vi "Stimulus trigger logic-Funct protocols.vi"(8 "Start trigger not fired":bool, 9 "Trigger lines value":T1, 10 "Tick Count(Ticks) in":u32, 11 "Stimulus Trigger Setup":T2={"Trigger period in live protocols (80MHz Cycles)"=510000000, "Pulse width in live protocols (80MHz Cycles)"=80000000, "Enable stimulus in live protocols"=FALSE, "Trigger delay in funct. protocols (80MHz Cycles)"=0, "Pulse width in funct. protocols (80MHz Cycles)"=400000, "Enable stimulus in funct. protocols"=FALSE}) -> (0 "Start trigger not fired":bool, 2 "Tick Count(Ticks) out":u32, 5 "Output value":bool)   [LabVIEW 2020]
uses:
  <vilib>/eio/EIONode/EIONode.xnode
  <vilib>/rvi/eio/common/nirviEmuTemplateMethod_errors.vi
  FPGA Typedefs/Stimulus trigger delays cluster.ctl
  FPGA Typedefs/PXI Trigger lines value cluster.ctl
panel:
  out "RAW counter VI":u32
  # "Limited to 53.5 sec (if U32)"
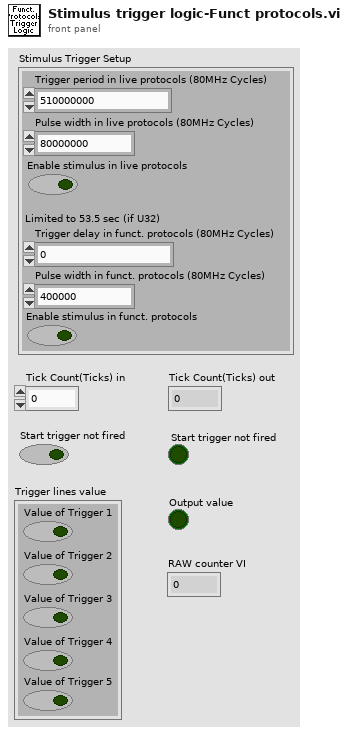
[diagram p1: front panel]
types:
  T1 = typedef "PXI Trigger lines value cluster.ctl" = cluster{"Value of Trigger 1":bool, "Value of Trigger 2":bool, "Value of Trigger 3":bool, "Value of Trigger 4":bool, "Value of Trigger 5":bool}
  T2 = typedef "Stimulus trigger delays cluster.ctl" = cluster{"Trigger period in live protocols (80MHz Cycles)":u32, "Pulse width in live protocols (80MHz Cycles)":u32, "Enable stimulus in live protocols":bool, "Trigger delay in funct. protocols (80MHz Cycles)":u32, "Pulse width in funct. protocols (80MHz Cycles)":u32, "Enable stimulus in funct. protocols":bool}
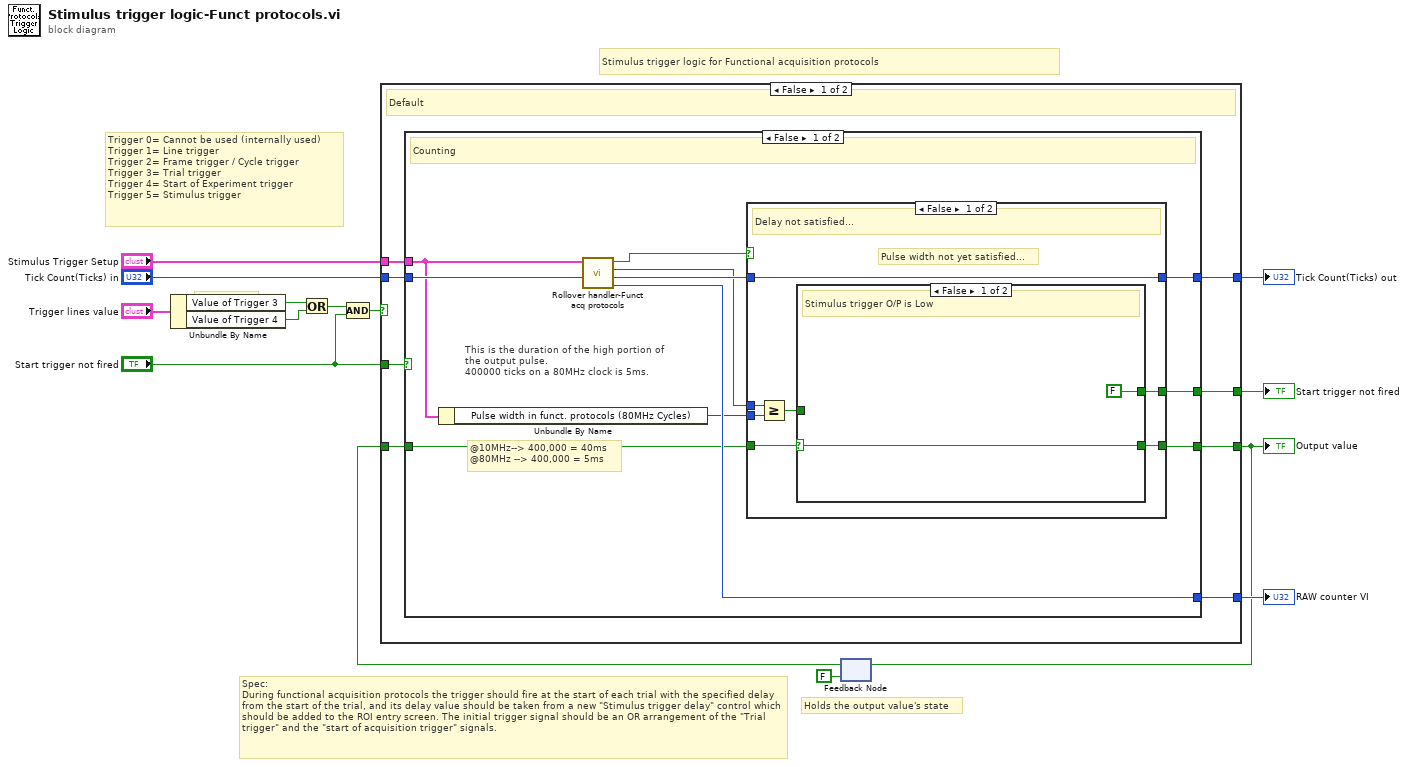
[diagram p0: block diagram]
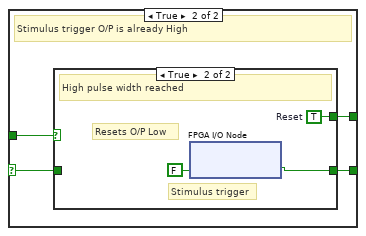
[diagram p2: hidden frame]
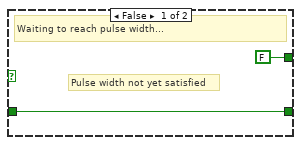
[diagram p3: hidden frame]
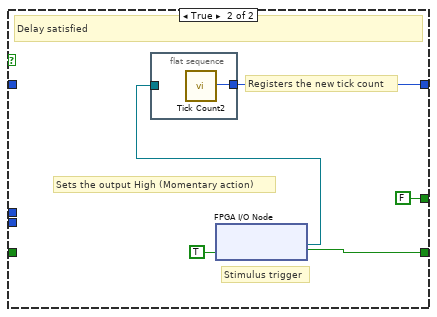
[diagram p4: hidden frame]
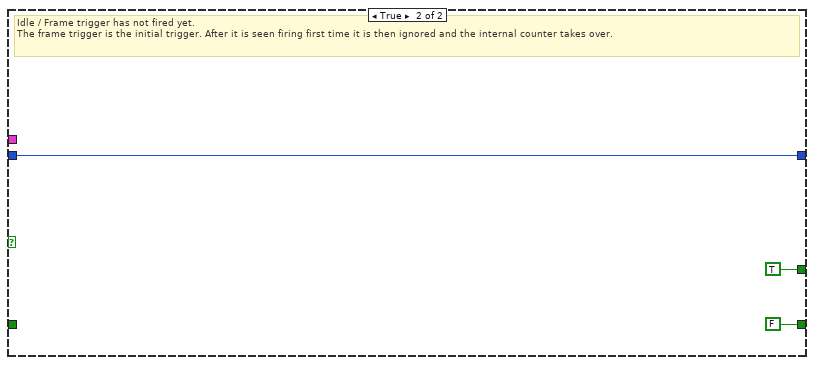
[diagram p5: hidden frame]
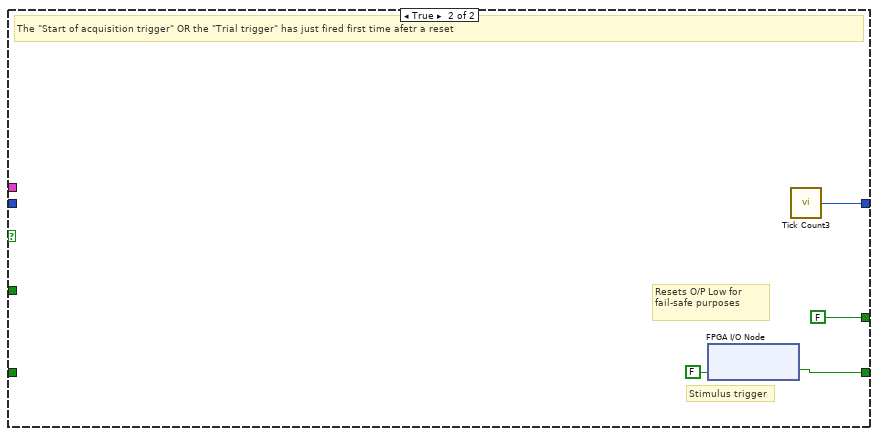
[diagram p6: hidden frame]
diagram:
  # "Holds the output value's state"
  # "Trigger 0= Cannot be used (internally used)\nTrigger 1= Line trigger\nTrigger 2= Frame trigger / Cycle trigger\nTrigger 3= Trial trigger\nTrigger 4= Start of Experiment trigger\nTrigger 5= Stimulus trigger"
  # "Trial trigger"
  # "Spec:\nDuring functional acquisition protocols the trigger should fire at the start of each trial with the specified delay from the start of the trial, and its delay value should be taken from a new \"Stimulus trigger delay\" control which should be added to the ROI entry screen. The initial trigger signal should be an OR arrangement of the \"Trial trigger\" and the \"start of acquisition trigger\" signals."
  # "Stimulus trigger logic for Functional acquisition protocols"
  n1 = Unbundle By Name("Trigger lines value") -> ("Value of Trigger 3"=w6:bool, "Value of Trigger 4"=w7:bool)
  n2 = Or(x=w6, y=w7) -> (x .or. y?=w5:bool)
  n3 = Compound Arithmetic op=AND(w5, "Start trigger not fired") -> (w9:bool)
  n4 = feedback #1(FALSE ("PXI_Trig0")) -> (w1:bool)
  n5 = case shown="False" w9 {
    tunnel: [w20 w61] -> w10
    tunnel: "Tick Count(Ticks) in" -> [w22 _]
    tunnel: [w18 FALSE ("Reset")] -> w12
    tunnel: "Start trigger not fired" -> [w21 _]
    tunnel: "Stimulus Trigger Setup" -> [w19 _]
    tunnel: [w17 w59] -> w2
    tunnel: [w16 _] -> w4
    tunnel: w1 -> [w15 _]
    frame False {
      # "Default"
      n6 = case shown="False" w21 {
        tunnel: w22 -> [w30 w58]
        tunnel: [w32 w58] -> w20
        tunnel: w19 -> [w26 _]
        tunnel: [w31 TRUE ("Reset")] -> w18
        tunnel: [w28 FALSE ("PXI_Trig0")] -> w17
        tunnel: [w27 _] -> w16
        tunnel: w15 -> [w25 _]
        frame False {
          # "This is the duration of the high portion of the output pulse.\n400000 ticks on a 80MHz clock is 5ms."
          # "@10MHz--> 400,000 = 40ms\n@80MHz --> 400,000 = 5ms"
          # "Counting"
          n7 = Unbundle By Name(w26) -> ("Pulse width in funct. protocols (80MHz Cycles)"=w24:u32)
          n8 = call "Rollover handler-Funct acq protocols.vi"("Tick Count Register in"=w30, "Stimulus Trigger Setup"=w26) -> ("Raw count"=w27:u32, "Tick Count Register out"=w29:u32, "Elapsed ticks count"=w23:u32, "Target reached"=w33:bool)  [unwired: 6 in]
          n9 = case shown="False" w33 {
            tunnel: w29 -> [w40 _]
            tunnel: [w40 w54] -> w32
            tunnel: [w38 w52] -> w28
            tunnel: w25 -> [w39 _]
            tunnel: [w37 FALSE ("Reset")] -> w31
            tunnel: w24 -> [w35 _]
            tunnel: w23 -> [w34 _]
            frame False {
              # "Pulse width not yet satisfied..."
              # "Delay not satisfied..."
              n10 = Greater Or Equal?(x=w34, y=w35) -> (x >= y?=w36:bool)
              n11 = case shown="False" w39 {
                selector: w39 -> [w42 w44]
                tunnel: [w42 w46] -> w38
                tunnel: w36 -> [_ w45]
                tunnel: [FALSE ("Reset") w43] -> w37
                frame False {
                  # "Stimulus trigger O/P is Low"
                }
                frame True {
                  # "Stimulus trigger O/P is already High"
                  n12 = case shown="True" w45 {
                    tunnel: [w48 w49] -> w46
                    tunnel: w44 -> [w48 _]
                    tunnel: [FALSE ("Reset") w50] -> w43
                    frame False {
                      # "Pulse width not yet satisfied"
                      # "Waiting to reach pulse width..."
                    }
                    frame True {
                      w50 = TRUE  # Reset
                      w49 = FALSE ("PXI_Trig0")
                      # "Resets O/P Low"
                      # "Stimulus trigger"
                      # "High pulse width reached"
                      n13 = xnode "FPGA I/O Node"("PXI_Trig5"=w49) -> ()  [unwired: 1 in, 1 out]
                    }
                  }
                }
              }
            }
            frame True {
              w52 = TRUE ("PXI_Trig0")
              # "Registers the new tick count"
              # "Sets the output High (Momentary action)"
              # "Stimulus trigger"
              # "Delay satisfied"
              n14 = flat-sequence {
                tunnel: [w55] -> w54
                tunnel: w51 -> [_]
                frame #0 {
                  n15 = call "Tick Count2"() -> ("Tick Count(Ticks)"=w55:u32)
                }
              }
              n16 = xnode "FPGA I/O Node"("PXI_Trig5"=w52) -> ("FPGA I/O Out"=w51:refnum<k21>)  [unwired: 1 in]
            }
          }
        }
        frame True {
          # "Idle / Frame trigger has not fired yet. \nThe frame trigger is the initial trigger. After it is seen firing first time it is then ignored and the internal counter takes over."
        }
      }
    }
    frame True {
      w59 = FALSE ("PXI_Trig0")
      # "Resets O/P Low for fail-safe purposes"
      # "Stimulus trigger"
      # "The \"Start of acquisition trigger\" OR the \"Trial trigger\" has just fired first time afetr a reset"
      n17 = xnode "FPGA I/O Node"("PXI_Trig5"=w59) -> ()  [unwired: 1 in, 1 out]
      n18 = call "Tick Count3"() -> ("Tick Count(Ticks)"=w61:u32)
    }
  }
  "Start trigger not fired" <- w12
  "Tick Count(Ticks) out" <- w10
  "Output value" <- w2
  "RAW counter VI" <- w4
  n19 = feedback-in #1(w2) -> ()
